vi "set_params.vi"(8 "error in (no error)":errorcluster caption="entrée d'erreur (pas d'erreur)", 11 "LinearSVR.lvclass 2":refnum<class "LinearSVR.lvclass">) -> (0 "error out":errorcluster caption="sortie d'erreur", 3 "LinearSVR.lvclass":refnum<class "LinearSVR.lvclass">)   [LabVIEW 2020, in "LinearSVR.lvclass"]
uses:
  LinearSVR.lvclass
  LinearSVR.lvclass/LinearSVR.ctl
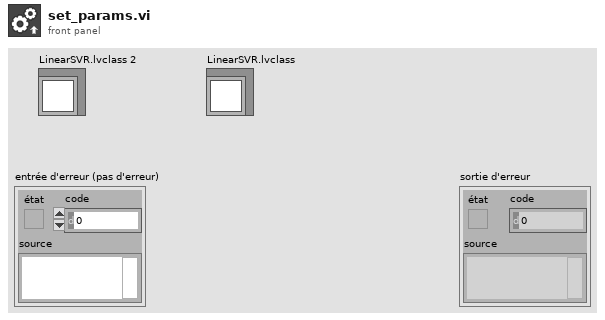
[diagram p1: front panel]
types:
  T1 = typedef "linear_svr_params.ctl" = cluster{"epsilon":dbl, "tol":dbl, "C":dbl, "loss":string, "fit_intercept":bool, "intercept_scaling":dbl, "dual":bool, "verbose":dbl, "random_state":dbl, "max_iter":dbl}
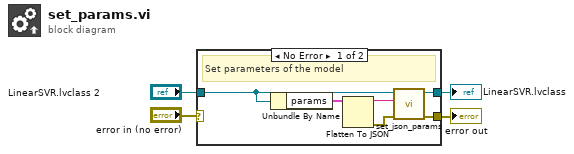
[diagram p0: block diagram]
diagram:
  n1 = case shown="No Error" "error in (no error)" {
    selector: "error in (no error)" -> [_ w12]
    tunnel: [w7 w12] -> w3
    tunnel: [w8 w11] -> w1
    tunnel: "LinearSVR.lvclass 2" -> [w5 w11]
    frame No Error {
      # "Set parameters of the model"
      n2 = Unbundle By Name(w5) -> ("params"=w10:T1)
      n3 = Flatten To JSON(anything=w10) -> (JSON string=w9:string, 11:w6:errorcluster)  [unwired: 2 in]
      n4 = call-dynamic "set_json_params.vi"("error in (no error)"=w6, "params"=w9, "Model en entrée"=w5) -> ("error out"=w7:errorcluster, "Model en sortie"=w8:refnum<class "LinearSVR.lvclass">)  [unwired: 7 in]
    }
    frame Error {
    }
  }
  "error out" <- w3
  "LinearSVR.lvclass" <- w1
